vi "Set_Tunnel_Speed.vi"(3 "Mode":T1, 5 "Tunnel Velocity m/s":dbl min=0.0 max=50.0 format="%.2f") -> (0 "Error String":string)   [LabVIEW 2010]
doc: "This is an example of using features of the VI Server as a client. It shows how you might browse from one or more applications that may be exporting data from one or more data stations. \n\nThe example shows how to query a server for its list of exported VIs, how to get references to the VIs, and how call them with the Call By Reference function."
uses:
  Sub VIs/ADAM Controls/Tunnel_speed_mode.ctl
  Sub VIs/ADAM Controls/Update_scan_value.ctl
  Sub VIs/ADAM Controls/Channel_State.ctl
  Sub VIs/ADAM Controls/Calib_type_ADAM.ctl
  Sub VIs/ADAM Controls/Module_type_ADAM.ctl
  Sub VIs/ADAM Controls/Ch_description_ADAM.ctl
  Sub VIs/ADAM Controls/Function_ADAM.ctl
  Sub VIs/ADAM Controls/Address.ctl
  Anemometry/Anemometry Sub Vis/Controls/Global_mode.ctl
  Anemometry/Anemometry Sub Vis/Globals/Preference_global.vi
  Anemometry/Anemometry Sub Vis/Globals/Trav_pos_global.vi
  Anemometry/Anemometry Sub Vis/Globals/Constants_global.vi
panel:
  in  "Set EnFlo Tun Speed":refnum<vi>
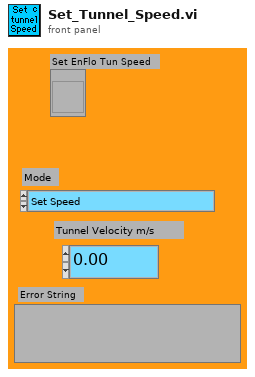
[diagram p1: front panel]
types:
  T1 = typedef "Tunnel_speed_mode.ctl" = enum16{"Set Speed", "Set Speed then wait", "Is tunnel speed allowable?"}
  T2 = typedef "Update_scan_value.ctl" = cluster{"Channel Name":string, "New Value":dbl}
  T3 = typedef "Channel_State.ctl" = enum16{"On", "Off", "Always On", "Always Off"}
  T4 = typedef "Calib_type_ADAM.ctl" = enum16{"Raw", "Bx + A", "Cx^2 + Bx + A", "Dx^3 + Cx^2 + Bx + A", "In Band", "Hi-Tec Q", "Hi-Tec M_dot", "Text"}
  T5 = typedef "Module_type_ADAM.ctl" = enum16{"4011", "4012", "4013", "4014", "4016", "4017", "4018", "4021", "4050", "4052", "4053", "4060", "4080", "5000", "5017", "5018", "5024", "5051", "5056", "5060", "6060", "Tracker", "WEST", "GILL", "JEM", "VICI", "Vaisala", "DRUCK", "Run VI Named:", "IR2100", "PPT", "Comparator", "VIRTUAL", "Hold Value", "Read A", "Read Ch", "Coded", "Client Info", "Web Client", "X10", "Test"}
  T6 = typedef "Ch_description_ADAM.ctl" = cluster{"Ch Name":string, "Type":T5, "Function":T7, "Ch State":T3, "Calibration type":T4, "A":dbl, "B":dbl, "C":dbl, "D":dbl, "Comments":string, "Address":T8, "String":string, "Duty":u16}
  T7 = typedef "Function_ADAM.ctl" = enum16{"Analogue Input", "Digital Input", "Event counter", "Event rate", "Analogue Output", "Digital Output", "Relay Output"}
  T8 = typedef "Address.ctl" = cluster{"Main":i32, "Ch.":i32, "Sub":i32, "Port Name":string}
  T9 = typedef "Global_mode.ctl" = enum16{"Read Global", "Load Global From File", "Write Global to File"}
  T10 = typedef "Server_Comms.ctl" = enum16{"Server Link Healthy", "Do Not Link To Server"}
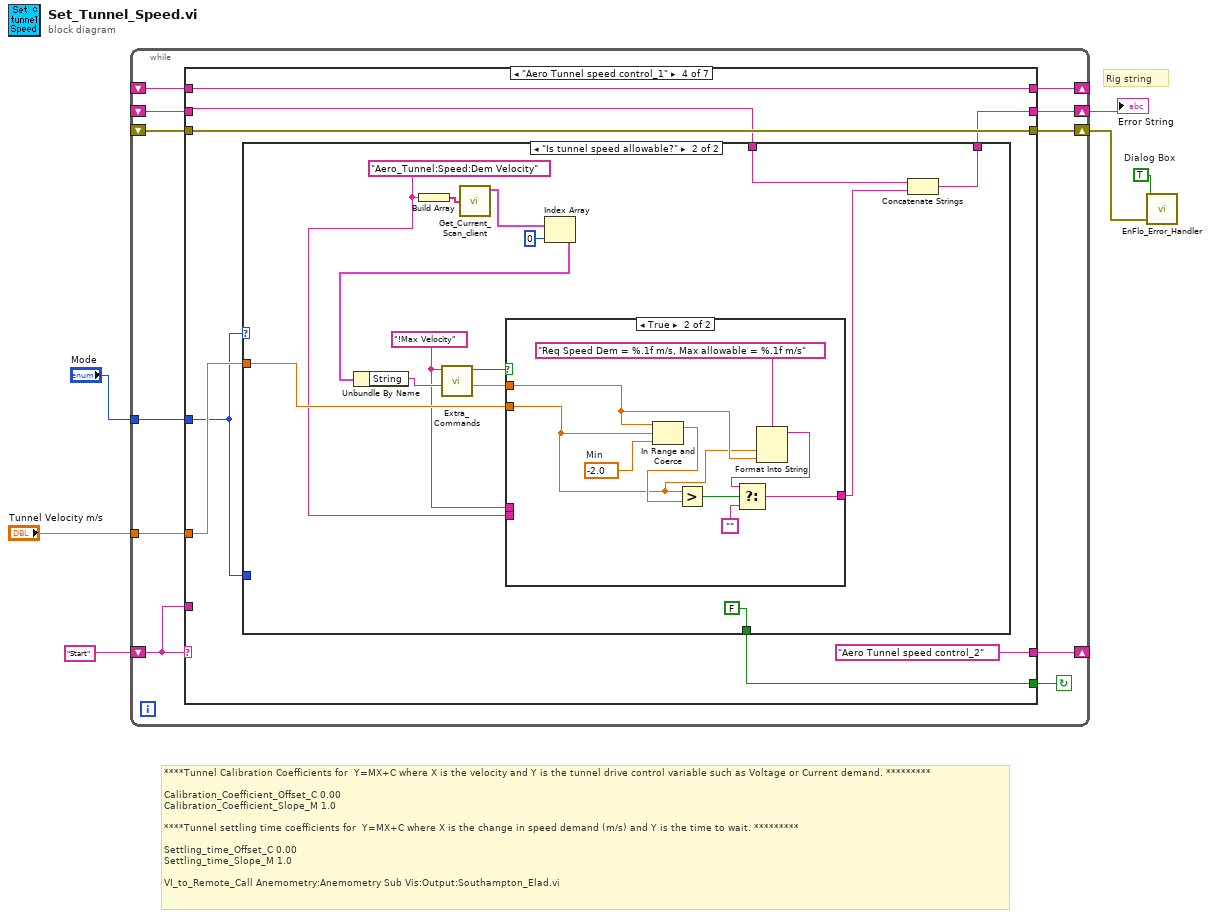
[diagram p0: block diagram]
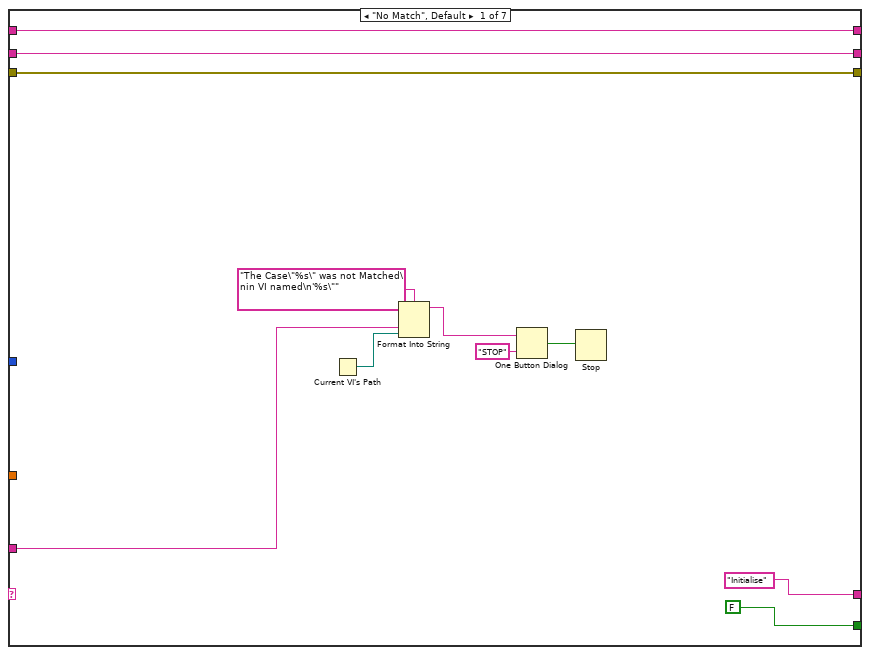
[diagram p2: hidden frame]
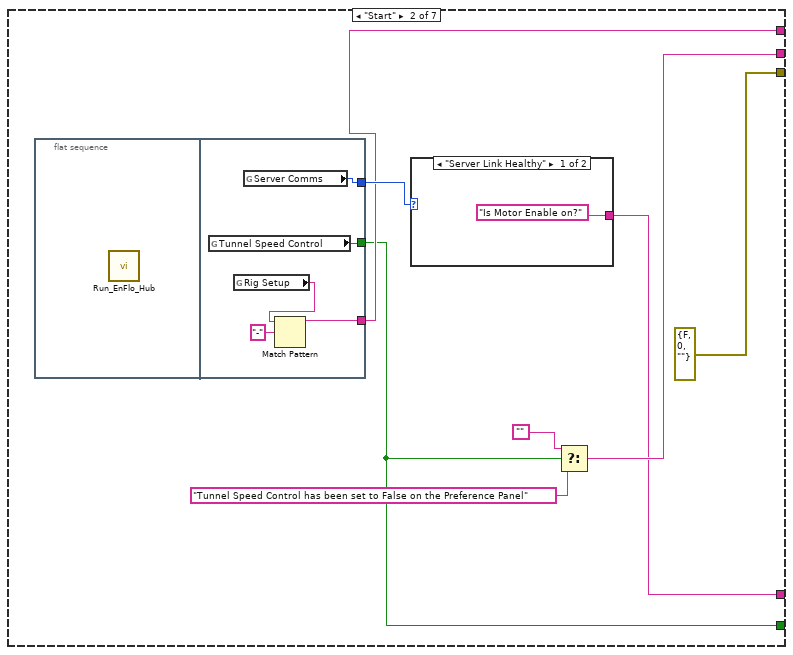
[diagram p3: hidden frame]
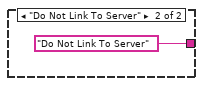
[diagram p4: hidden frame]
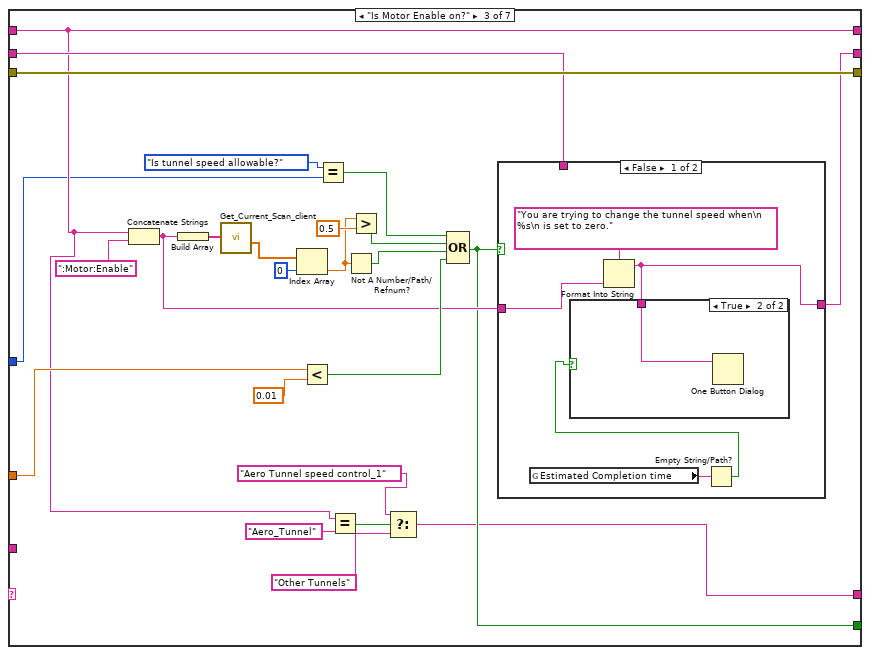
[diagram p5: hidden frame]
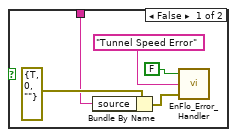
[diagram p6: hidden frame]
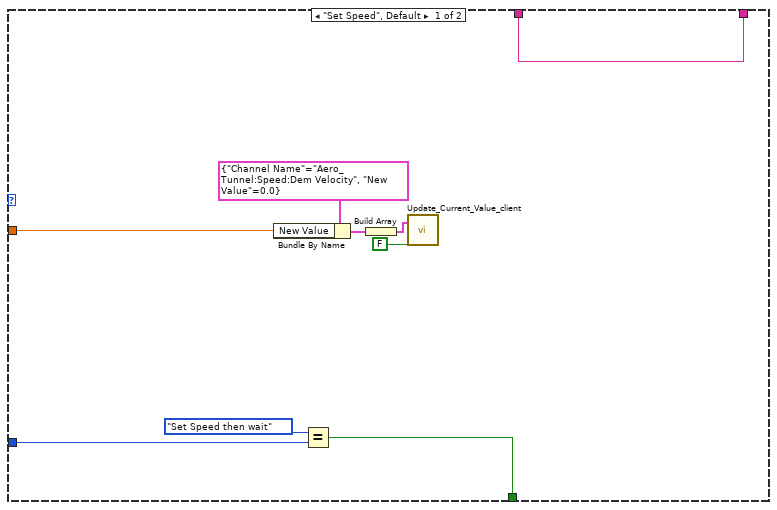
[diagram p8: hidden frame]
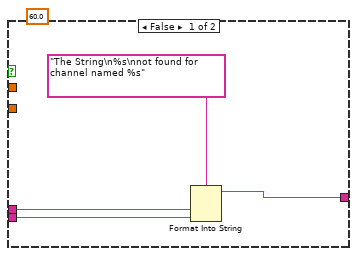
[diagram p9: hidden frame]
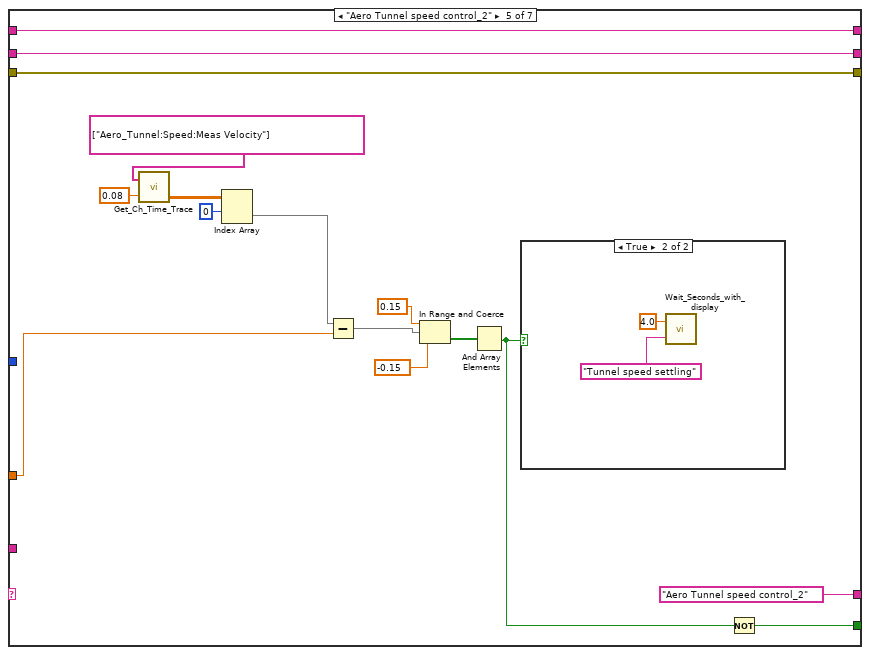
[diagram p10: hidden frame]
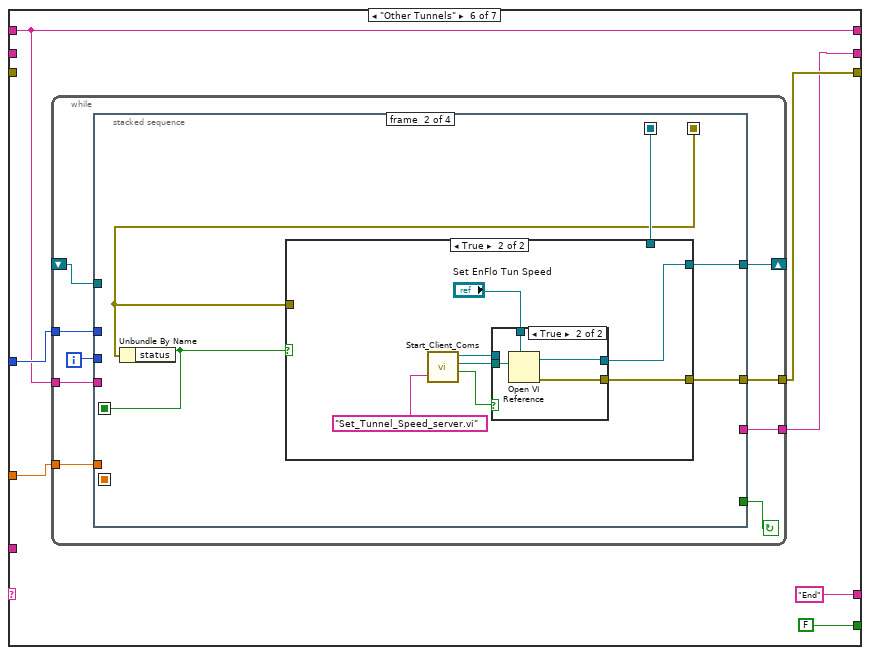
[diagram p12: hidden frame]
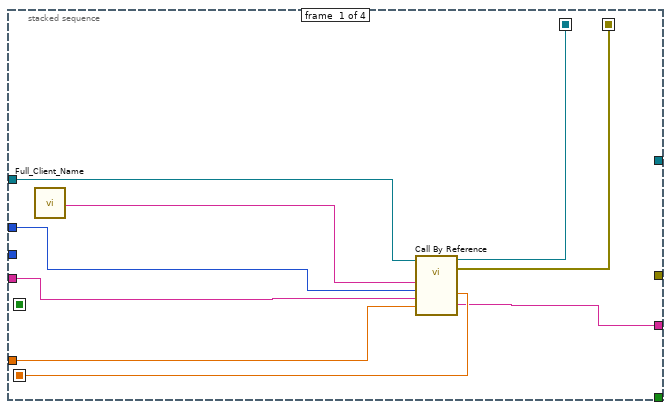
[diagram p13: hidden frame]
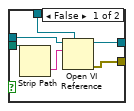
[diagram p15: hidden frame]
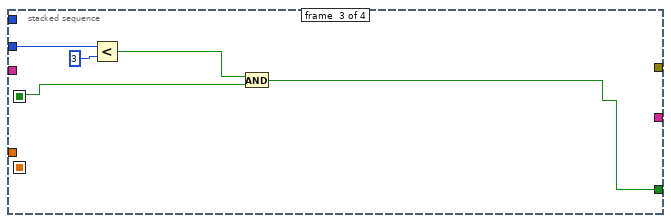
[diagram p16: hidden frame]
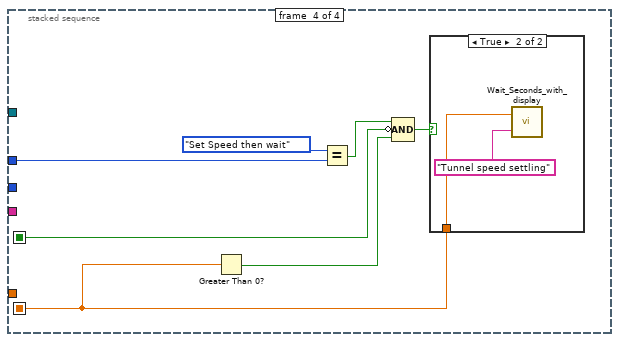
[diagram p17: hidden frame]
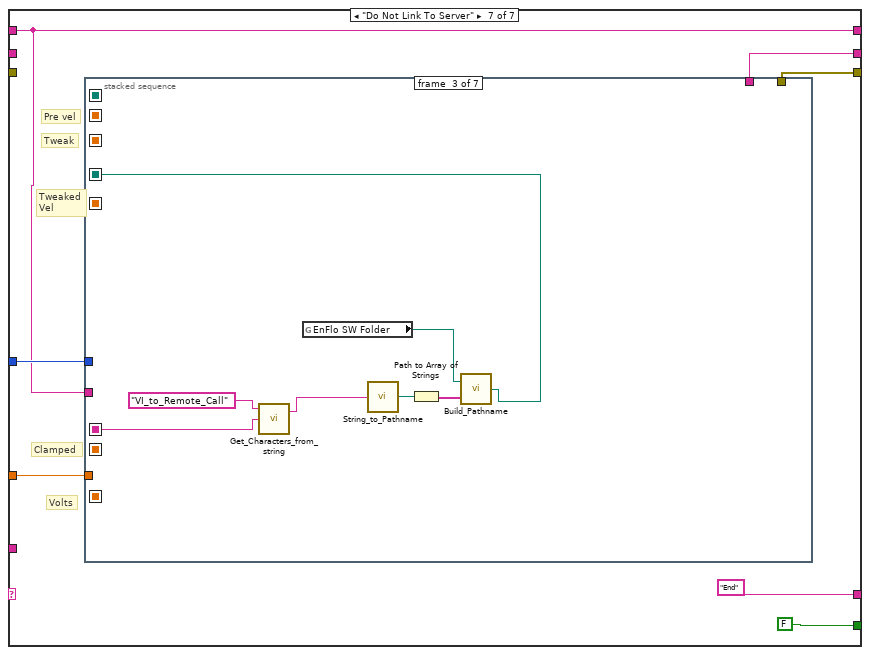
[diagram p19: hidden frame]
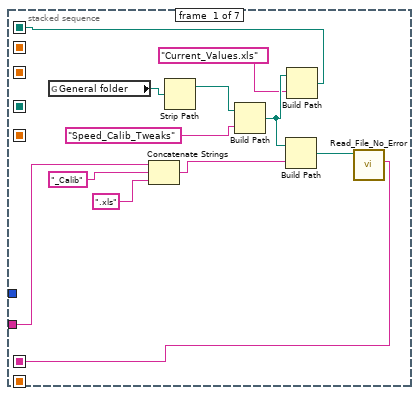
[diagram p20: hidden frame]
diagram:
  w6 = TRUE  # Dialog Box
  # "Rig string"
  # "****Tunnel Calibration Coefficients for  Y=MX+C where X is the velocity and Y is the tunnel drive control variable such as Voltage or Current demand. *********\n\nCalibration_Coefficient_Offset_C\t0.00\nCalibration_Coefficient_Slope_M\t1.0\n\n****Tunnel settling time coefficients for  Y=MX+C where X is the change in speed demand (m/s) and Y is the time to wait. *********\n\nSettling_time_Offset_C\t0.00\nSettling_time_Slope_M\t1.0\n\nVI_to_Remote_Call\tAnemometry:Anemometry Sub Vis:Output:Southampton_Elad.vi"
  n1 = while {
    shift-left: "Start" -> [w16]
    shift-right: [w17] -> _
    shift-right: [w15] -> w4
    shift-left: _ -> [w14]
    shift-right: [w13] -> w3
    shift-left: _ -> [w8]
    tunnel: "Mode" -> [w12]
    tunnel: "Tunnel Velocity m/s" -> [w11]
    shift-right: [w10] -> _
    shift-left: _ -> [w9]
    stop <- w7 continue-if-true
    n2 = case shown="\"Aero Tunnel speed control_1\"" w16 {
      tunnel: [FALSE w33 w53 w84 w125 FALSE ("Tunnel Speed Control") FALSE] -> w7
      tunnel: ["Initialise" w29 w47 "Aero Tunnel speed control_2" ("f") "Aero Tunnel speed control_2" ("f") "End" ("f") "End"] -> w17
      tunnel: w16 -> [w23 _ _ _ _ _ _]
      tunnel: [w20 w31 w55 w81 w138 w146 w208] -> w15
      tunnel: w14 -> [w20 _ w54 w82 w138 _ _]
      tunnel: [w18 errorcluster {"status"=FALSE, "code"=0, "source"=""} ("error out") w57 w85 w137 w147 w207] -> w13
      tunnel: w12 -> [_ _ w45 w83 _ w149 w210]
      tunnel: w11 -> [_ _ w58 w88 w131 w148 w209]
      tunnel: [w19 w34 w51 w86 w139 w145 w206] -> w10
      tunnel: w9 -> [w19 _ w51 w86 w139 w145 w206]
      tunnel: w8 -> [w18 _ w57 w85 w137 _ _]
      frame "No Match", Default {
        n3 = Current VI's Path() -> (path=w22:path)
        n4 = Format Into String(format string="The Case\"%s\" was not Matched\nin VI named\n'%s\"" ("Format String"), w23, w22) -> (resulting string=w26:string)  [unwired: 2 in, 1 out]
        n5 = One Button Dialog(message=w26, button name ("OK")="STOP") -> (true=w24:bool)
        n6 = Stop(stop? (T)=w24) -> ()
      }
      frame "Start" {
        n7 = flat-sequence {
          tunnel: [w43] -> w36
          tunnel: [w42] -> w33
          tunnel: [w39] -> w34
          frame #0 {
            n8 = call "Run_EnFlo_Hub.vi"() -> ()  [unwired: 8 out]
          }
          frame #1 {
            n9 = global read "Preference_global.vi" "Tunnel Speed Control"() -> (w42:bool)
            n10 = global read "Preference_global.vi" "Rig Setup"() -> (w41:string)
            n11 = global read "Preference_global.vi" "Server Comms"() -> (w43:T10)
            n12 = Match Pattern(string=w41, regular expression="-") -> (before substring=w39:string)  [unwired: 4 out]
          }
        }
        n13 = case shown="\"Server Link Healthy\"" w36 {
          tunnel: ["Is Motor Enable on?" "Do Not Link To Server"] -> w29
          frame "Server Link Healthy" {
          }
          frame "Do Not Link To Server" {
          }
        }
        n14 = Select(t="", s=w33, f="Tunnel Speed Control has been set to False on the Preference Panel" ("Error String")) -> (s? t:f=w31:string)
      }
      frame "Is Motor Enable on?" {
        n15 = Concatenate Strings(w51, ":Motor:Enable" ("string")) -> (w56:string)
        n16 = Build Array(w56) -> (w60:string[])
        n17 = call "Get_Current_Scan_client.vi"("ADAM Ch Names"=w60) -> ("Numerical Values"=w61:dbl[])  [unwired: 3 out]
        n18 = Index Array(array=w61, index=0) -> (element=w63:dbl)
        n19 = Less?(x=w58, y=0.01) -> (x < y?=w68:bool)
        n20 = Equal?(x=Tunnel_speed_mode."Is tunnel speed allowable?" ("Mode"), y=w45) -> (x = y?=w44:bool)
        n21 = Equal?(x=w51, y="Aero_Tunnel") -> (x = y?=w50:bool)
        n22 = Not A Number/Path/Refnum?(number/path/refnum=w63) -> (NaN/Path/Refnum?=w65:bool)
        n23 = Greater?(x=w63, y=0.5) -> (0:w66:bool)
        n24 = Select(t="Aero Tunnel speed control_1", s=w50, f="Other Tunnels") -> (s? t:f=w47:string)
        n25 = Compound Arithmetic op=OR(w44, w66, w65, w68) -> (w53:bool)
        n26 = case shown="False" w53 {
          tunnel: w56 -> [w72 _]
          tunnel: [w69 w80] -> w55
          tunnel: w54 -> [_ w80]
          frame False {
            n27 = global read "Trav_pos_global.vi" "Estimated Completion time"() -> (w71:string)
            n28 = Format Into String(format string="You are trying to change the tunnel speed when\n %s\n is set to zero.", w72) -> (resulting string=w69:string)  [unwired: 2 in, 1 out]
            n29 = Empty String/Path?(string/path=w71) -> (empty?=w70:bool)
            n30 = case shown="True" w70 {
              tunnel: w69 -> [w75 w79]
              frame False {
                n31 = Bundle By Name(cluster=errorcluster {"status"=TRUE, "code"=0, "source"=""} ("error in (no error)"), "source"=w75) -> (w76:errorcluster)
                n32 = call "EnFlo_Error_Handler.vi"("error in (no error)"=w76, "Error Type"="Tunnel Speed Error", "Dialog Box (T)"=FALSE) -> ()  [unwired: 3 out]
              }
              frame True {
                n33 = One Button Dialog(message=w79) -> ()  [unwired: 2 out]
              }
            }
          }
          frame True {
          }
        }
      }
      frame "Aero Tunnel speed control_1" {
        n34 = case shown="\"Is tunnel speed allowable?\"" w83 {
          tunnel: w88 -> [w93 w106]
          tunnel: [w90 FALSE] -> w84
          tunnel: w83 -> [w91 _]
          tunnel: w82 -> [w89 w101]
          tunnel: [w89 w100] -> w81
          frame "Set Speed", Default {
            n35 = Bundle By Name(cluster=T2 {"Channel Name"="Aero_Tunnel:Speed:Dem Velocity", "New Value"=0.0} ("Update Scan Value Cluster"), "New Value"=w93) -> (w95:T2)
            n36 = Equal?(x=Tunnel_speed_mode."Set Speed then wait" ("Mode"), y=w91) -> (x = y?=w90:bool)
            n37 = Build Array(w95) -> (w96:T2[])
            n38 = call "Update_Current_Value_client.vi"("Don't Bother with check?"=FALSE, "Update array in"=w96) -> ()
          }
          frame "Is tunnel speed allowable?" {
            w105 = "!Max Velocity" ("Command")
            w104 = "Aero_Tunnel:Speed:Dem Velocity"
            n39 = Build Array(w104) -> (w99:string[])
            n40 = call "Get_Current_Scan_client.vi"("ADAM Ch Names"=w99) -> ("Ch Description Array"=w98:T6[])  [unwired: 1 in, 2 out]
            n41 = Index Array(array=w98, index=0 ("Index")) -> (element=w111:T6)
            n42 = Unbundle By Name(w111) -> ("String"=w110:string)
            n43 = call "Extra_Commands.vi"("String to Search"=w110, "Command"=w105) -> ("Numeric Value"=w107:dbl, "Command Found"=w108:bool)  [unwired: 1 in, 3 out]
            n44 = case shown="True" w108 {
              tunnel: w105 -> [w115 _]
              tunnel: w104 -> [w114 _]
              tunnel: [w112 w120] -> w102
              tunnel: w107 -> [_ w117]
              tunnel: w106 -> [_ w116]
              frame False {
                (unwired) 60.0 ("Numeric Value")
                n45 = Format Into String(format string="The String\n%s\nnot found for channel named %s" ("Format String"), w115, w114) -> (resulting string=w112:string)  [unwired: 2 in, 1 out]
              }
              frame True {
                w124 = -2.0  # Min
                n46 = In Range and Coerce(upper limit=w117, x=w116, lower limit=w124) -> (coerced(x)=w118:dbl)  [unwired: 1 out]
                n47 = Greater?(x=w116, y=w118) -> (0:w119:bool)
                n48 = Format Into String(format string="Req Speed Dem = %.1f m/s, Max allowable = %.1f m/s", w116, w117) -> (resulting string=w122:string)  [unwired: 2 in, 1 out]
                n49 = Select(t=w122, s=w119, f="") -> (s? t:f=w120:string)
              }
            }
            n50 = Concatenate Strings(w101, w102) -> (w100:string)
          }
        }
      }
      frame "Aero Tunnel speed control_2" {
        n51 = call "Get_Ch_Time_Trace.vi"("Desired Ch Names"=string[] ["Aero_Tunnel:Speed:Meas Velocity"] ("ADAM Ch Names"), "History Length (mins)"=0.08) -> ("Output array"=w134:dbl[][])  [unwired: 2 out]
        n52 = Index Array(array=w134, index (row)=0) -> (element=w132:dbl[])  [unwired: 1 in]
        n53 = Subtract(x=w132, y=w131) -> (x-y=w128:dbl[])
        n54 = In Range and Coerce(upper limit=0.15, x=w128, lower limit=-0.15) -> (In Range?=w127:bool[])  [unwired: 1 out]
        n55 = And Array Elements(Boolean array=w127) -> (logical AND=w126:bool)
        n56 = case shown="True" w126 {
          frame False {
          }
          frame True {
            n57 = call "Wait_Seconds_with_display.vi"("Message"="Tunnel speed settling", "Seconds to wait"=4.0) -> ()  [unwired: 2 out]
          }
        }
        n58 = Not(x=w126) -> (.not. x?=w125:bool)
      }
      frame "Other Tunnels" {
        n59 = while {
          tunnel: w149 -> [w153]
          tunnel: w148 -> [w154]
          tunnel: [w155] -> w147
          shift-left: _ -> [w150]
          shift-right: [w158] -> _
          tunnel: [w152] -> w146
          tunnel: w145 -> [w151]
          i -> [w157]
          stop <- w156 continue-if-true
          n60 = stacked-sequence {
            seq-local: [w166 _ _ _] -> [_ w171 _ _]
            seq-local: [w165 _ _ _] -> [_ w169 _ _]
            seq-local: [_ w170 _ _] -> [_ _ w193 w198]
            seq-local: [w162 _ _ _] -> [_ _ _ w202]
            tunnel: w150 -> [w167 _ _ _]
            tunnel: [_ w172 _ _] -> w158
            tunnel: w157 -> [_ _ w194 _]
            tunnel: [_ _ w192 _] -> w156
            tunnel: [_ w168 _ _] -> w155
            tunnel: w154 -> [w163 _ _ _]
            tunnel: w153 -> [w159 _ _ w203]
            tunnel: [w161 _ _ _] -> w152
            tunnel: w151 -> [w160 _ _ _]
            frame #0 {
              n61 = call "Full_Client_Name.vi"() -> ("Client Name"=w164:string)
              n62 = call-by-ref "?"(reference=w167, "Tunnel Velocity m/s"=w163, "Rig Name"=w160, "Mode"=w159, "Client Name"=w164) -> (reference out=w166:refnum<vi>, error out=w165:errorcluster, "Error String"=w161:string, "Settling Time (s)"=w162:dbl)  [unwired: 1 in, 1 out]
            }
            frame #1 {
              n63 = Unbundle By Name(w169) -> ("status"=w170:bool)
              n64 = case shown="True" w170 {
                tunnel: [w173 w177] -> w172
                tunnel: w171 -> [w173 _]
                tunnel: [w174 w176] -> w168
                tunnel: w169 -> [w174 _]
                frame False {
                }
                frame True {
                  n65 = call "Start_Client_Coms.vi"("VI name to run on server"="Set_Tunnel_Speed_server.vi") -> ("LabVIEW application reference"=w179:refnum<vi>, "Checked VI name"=w180:path, "Local Call"=w178:bool)  [unwired: 1 in, 1 out]
                  n66 = case shown="True" w178 {
                    tunnel: [w186 w191] -> w177
                    tunnel: "Set EnFlo Tun Speed" -> [w184 w190]
                    tunnel: w180 -> [w183 w189]
                    tunnel: w179 -> [w182 _]
                    tunnel: [w185 w188] -> w176
                    frame False {
                      n67 = Strip Path(path=w183) -> (name=w187:string)  [unwired: 1 out]
                      n68 = Open VI Reference(type specifier VI Refnum (for type only)=w184, application reference (local)=w182, vi path=w187) -> (vi reference=w186:refnum<vi>, error out=w185:errorcluster)  [unwired: 1 in, 2 out]
                    }
                    frame True {
                      n69 = Open VI Reference(type specifier VI Refnum (for type only)=w190, vi path=w189) -> (vi reference=w191:refnum<vi>, error out=w188:errorcluster)  [unwired: 1 in, 3 out]
                    }
                  }
                }
              }
            }
            frame #2 {
              n70 = Less?(x=w194, y=3) -> (x < y?=w196:bool)
              n71 = And(x=w196, y=w193) -> (x .and. y?=w192:bool)
            }
            frame #3 {
              n72 = Greater Than 0?(x=w202) -> (x > 0?=w197:bool)
              n73 = Equal?(x=Tunnel_speed_mode."Set Speed then wait" ("Mode"), y=w203) -> (x = y?=w200:bool)
              n74 = Compound Arithmetic op=AND(w200, invert w198, w197) -> (w199:bool)
              n75 = case shown="True" w199 {
                tunnel: w202 -> [_ w204]
                frame False {
                }
                frame True {
                  n76 = call "Wait_Seconds_with_display.vi"("Message"="Tunnel speed settling", "Seconds to wait"=w204) -> ()  [unwired: 2 out]
                }
              }
            }
          }
        }
      }
      frame "Do Not Link To Server" {
        # "Clamped"
        # "Pre vel"
        # "Tweak"
        # "Tweaked\nVel"
        # "Volts"
        n77 = stacked-sequence {
          seq-local: [w216 _ _ _ _ _ _] -> [_ w235 w241 w249 w265 w324 _]
          seq-local: [_ _ w236 _ _ _ _] -> [_ _ _ _ w269 _ _]
          seq-local: [_ _ _ w245 _ _ _] -> [_ _ _ _ w264 _ w337]
          seq-local: [_ _ _ w248 _ _ _] -> [_ _ _ _ w267 w319 _]
          seq-local: [_ _ _ _ w266 _ _] -> [_ _ _ _ _ w318 _]
          seq-local: [_ _ _ w250 _ _ _] -> [_ _ _ _ _ _ w343]
          seq-local: [w213 _ _ _ _ _ _] -> [_ _ _ _ _ _ w345]
          seq-local: [_ w226 _ _ _ _ _] -> [_ _ _ w243 _ _ w342]
          tunnel: w209 -> [_ w227 _ _ _ _ _]
          tunnel: w206 -> [w218 _ _ w258 _ _ w339]
          tunnel: w210 -> [_ _ _ _ w268 w313 _]
          tunnel: [_ w225 _ _ _ _ _] -> w208
          tunnel: [_ _ _ _ w263 _ _] -> w207
          frame #0 {
            n78 = global read "Constants_global.vi" "General folder"() -> (w223:path)
            n79 = Concatenate Strings(w218, "_Calib" ("Substring"), ".xls" ("string")) -> (w220:string)
            n80 = Strip Path(path=w223) -> (stripped path=w222:path)  [unwired: 1 out]
            n81 = Build Path(base path=w222, name or relative path="Speed_Calib_Tweaks" ("Input Element")) -> (appended path=w215:path)
            n82 = Build Path(base path=w215, name or relative path=w220) -> (appended path=w217:path)
            n83 = Build Path(base path=w215, name or relative path="Current_Values.xls") -> (appended path=w213:path)
            n84 = call "Read_File_No_Error.vi"("Filename"=w217) -> ("string"=w216:string)  [unwired: 2 in, 7 out]
          }
          frame #1 {
            w229 = -2.0  # Min
            n85 = call "Get_value_from_string.vi"("Input string"=w235, "Variable name"="Maximum_Allowable_Tunnel_Speed") -> ("Value"=w228:dbl)  [unwired: 1 in, 1 out]
            n86 = In Range and Coerce(upper limit=w228, x=w227, lower limit=w229) -> (coerced(x)=w226:dbl)  [unwired: 1 out]
            n87 = Greater?(x=w227, y=w228) -> (0:w230:bool)
            n88 = Format Into String(format string="Req Speed Dem = %.1f m/s, Max allowable = %.1f m/s", w227, w228) -> (resulting string=w232:string)  [unwired: 2 in, 1 out]
            n89 = Select(t=w232, s=w230, f="") -> (s? t:f=w225:string)
          }
          frame #2 {
            n90 = call "Get_Characters_from_string.vi"("Input string"=w241, "Variable name"="VI_to_Remote_Call") -> ("Value"=w239:string)  [unwired: 1 in, 1 out]
            n91 = global read "Constants_global.vi" "EnFlo SW Folder"() -> (w237:path)
            n92 = call "String_to_Pathname.vi"("Input String"=w239) -> ("path"=w240:path)
            n93 = Path to Array of Strings(0:w240) -> (2:w238:string[])  [unwired: 1 out]
            n94 = call "Build_Pathname.vi"("Output Array"=w238, "Pathname"=w237) -> ("Appended path"=w236:path)
          }
          frame #3 {
            w256 = FALSE  # Tunnel Heated?
            n95 = local write "Tunnel Velocity m/s"(w243) -> ()
            n96 = call "Add_to_speed_calib_file.vi"("Desired Velocity"=w243, "Tunnel Heated?"=w256, "Rig Name"=w258, "Mode"=enum16{"Add Row", "Get Error Value"}."Get Error Value") -> ("Tweaked Demand"=w248:dbl, "Calib Tweak %"=w250:dbl)  [unwired: 2 in]
            n97 = Less?(x=w248, y=0.01) -> (x < y?=w246:bool)
            n98 = call "Get_value_from_string.vi"("Input string"=w249, "Variable name"="Calibration_Coefficient_Offset_C") -> ("Value"=w251:dbl)  [unwired: 1 in, 1 out]
            n99 = call "Get_value_from_string.vi"("Input string"=w249, "Variable name"="Calibration_Coefficient_Slope_M") -> ("Value"=w253:dbl)  [unwired: 1 in, 1 out]
            n100 = Multiply(x=w253, y=w248) -> (x*y=w252:dbl)
            n101 = Add(x=w251, y=w252) -> (x+y=w244:dbl)
            n102 = case shown="False" w246 {
              tunnel: w249 -> [_ w261]
              tunnel: [w259 w260] -> w245
              tunnel: w244 -> [w259 _]
              frame False {
              }
              frame True {
                n103 = call "Get_value_from_string.vi"("Input string"=w261, "Variable name"="Zero_Velocity_Output_Voltage") -> ("Value"=w260:dbl)  [unwired: 1 in, 1 out]
              }
            }
          }
          frame #4 {
            n104 = while {
              tunnel: w269 -> [w279]
              tunnel: w268 -> [w278]
              tunnel: w267 -> [w277]
              tunnel: [w276] -> w266
              shift-right: [w274] -> _
              shift-left: _ -> [w273]
              tunnel: [w272] -> w263
              tunnel: w265 -> [w271]
              tunnel: w264 -> [w270]
              stop <- TRUE stop-if-true
              n105 = case shown="\"Set Speed then wait\", Default" w278 {
                tunnel: w279 -> [_ w299]
                tunnel: w277 -> [_ w286]
                tunnel: [w281 w288] -> w276
                tunnel: [w281 w286] -> w274
                tunnel: w273 -> [w281 w287]
                tunnel: [errorcluster {"status"=FALSE, "code"=0, "source"=""} ("error out") w282] -> w272
                tunnel: w271 -> [_ _]
                tunnel: w270 -> [_ w285]
                frame "Is tunnel speed allowable?" {
                }
                frame "Set Speed then wait", Default {
                  n106 = Open VI Reference(type specifier VI Refnum (for type only)=refnum<vi> refnum, vi path=w299) -> (vi reference=w297:refnum<vi>, error out=w296:errorcluster)  [unwired: 1 in, 3 out]
                  n107 = property class="VI Interface Type 1"(reference=w297, error in=w296) -> (reference out=w294:refnum<vi>, error out=w295:errorcluster, "Front Panel.Open"=w293:bool)
                  n108 = case shown="False" w293 {
                    tunnel: w295 -> [w304 w307]
                    tunnel: w294 -> [w303 w308]
                    tunnel: [w302 w308] -> w292
                    tunnel: [w301 w307] -> w291
                    tunnel: [0.0 ("Tweaked Demand") w306] -> w288
                    tunnel: w287 -> [_ w306]
                    frame False {
                      n109 = property class="VI Interface Type 1"(reference=w303, error in=w304, "Front Panel.Open"=TRUE ("Front Panel Window:Open")) -> (reference out=w302:refnum<vi>, error out=w301:errorcluster)
                    }
                    frame True {
                    }
                  }
                  n110 = call-by-ref "?"(reference=w292, error in=w291, "Demand"=w285) -> (reference out=w289:refnum<vi>, error out=w290:errorcluster, "error out"=w283:errorcluster)
                  n111 = Close Reference(reference=w289, error in (no error)=w290) -> (error out=w284:errorcluster)
                  n112 = Select(t=w284, s=w284, f=w283) -> (s? t:f=w282:errorcluster)
                }
              }
            }
          }
          frame #5 {
            n113 = Subtract(x=w318, y=w319) -> (x-y=w317:dbl)
            n114 = Absolute Value(x=w317) -> (abs(x)=w311:dbl)
            n115 = call "Get_value_from_string.vi"("Input string"=w324, "Variable name"="Settling_time_Offset_C") -> ("Value"=w320:dbl)  [unwired: 1 in, 1 out]
            n116 = call "Get_value_from_string.vi"("Input string"=w324, "Variable name"="Settling_time_Slope_M") -> ("Value"=w322:dbl)  [unwired: 1 in, 1 out]
            n117 = Multiply(x=w322, y=w311) -> (x*y=w321:dbl)
            n118 = Add(x=w320, y=w321) -> (x+y=w312:dbl)
            n119 = Greater?(x=w311, y=0.05) -> (0:w309:bool)
            n120 = Equal?(x=Tunnel_speed_mode."Set Speed then wait" ("Mode"), y=w313) -> (x = y?=w315:bool)
            n121 = Compound Arithmetic op=AND(w309, w315) -> (w314:bool)
            n122 = case shown="False" w314 {
              tunnel: w312 -> [_ w326]
              frame False {
              }
              frame True {
                n123 = call "Wait_Seconds_with_display.vi"("Message"="Tunnel speed settling", "Seconds to wait"=w326) -> ()  [unwired: 2 out]
              }
            }
          }
          frame #6 {
            n124 = Concatenate Strings(w339, ":Speed:Dem_Voltage" ("string")) -> (w334:string)
            n125 = Bundle By Name(cluster=T2 {"Channel Name"="", "New Value"=0.0} ("Update Scan Value Cluster"), "Channel Name"=w334, "New Value"=w337) -> (w340:T2)
            n126 = call "Value_to_string.vi"("Value"=w343, "Label for value"="Calib Tweak") -> ("Output string"=w348:string)  [unwired: 1 in]
            n127 = call "Value_to_string.vi"("Value"=w342, "Label for value"="Velocity Demand") -> ("Output string"=w347:string)  [unwired: 1 in]
            n128 = Concatenate Strings(w348, w347) -> (w346:string)
            n129 = Bundle By Name(cluster=T6 {"Ch Name"="", "Type"=enum."4011", "Function"=enum."Analogue Input", "Ch State"=enum."On", "Calibration type"=enum."Raw", "A"=0.0, "B"=0.0, "C"=0.0, "D"=0.0, "Comments"="", "Address"={"Main"=0, "Ch."=0, "Sub"=0, "Port Name"=""}, "String"="", "Duty"=0} ("Ch Discription"), "Ch Name"=w334, "Type"=Module_type_ADAM."Hold Value", "Calibration type"=Calib_type_ADAM."Raw", "Ch State"=Channel_State."On") -> (w328:T6)
            n130 = call "Write_File_Simple.vi"("append to file? (new file:F)"=FALSE, "character string"=w346, "file path"=w345) -> ()  [unwired: 2 out]
            n131 = Build Array(w340) -> (w330:T2[])
            n132 = Build Array(w328) -> (w329:T6[])
            n133 = call "Read_Write_Local_table.vi"("Mode"=Global_mode."Write Global to File", "Ch Values in"=w330, "Channels Descriptions In"=w329) -> ()  [unwired: 3 out]
          }
        }
      }
    }
  }
  "Error String" <- w4
  n134 = call "EnFlo_Error_Handler.vi"("error in (no error)"=w3, "Dialog Box (T)"=w6) -> ()  [unwired: 1 in, 3 out]
